vi "setValue.vi"(8 "error in (no error)":errorcluster, 10 "Time Stamp":timestamp, 11 "tBSONTimestamp in":refnum<class "tBSONTimestamp.lvclass">) -> (0 "error out":errorcluster, 3 "tBSONTimestamp out":refnum<class "tBSONTimestamp.lvclass">)   [LabVIEW 2013, in "BSON.lvlib" / "tBSONTimestamp.lvclass"]
uses:
  tBSONTimestamp.lvclass
  tBSONTimestamp.lvclass/tBSONTimestamp.ctl
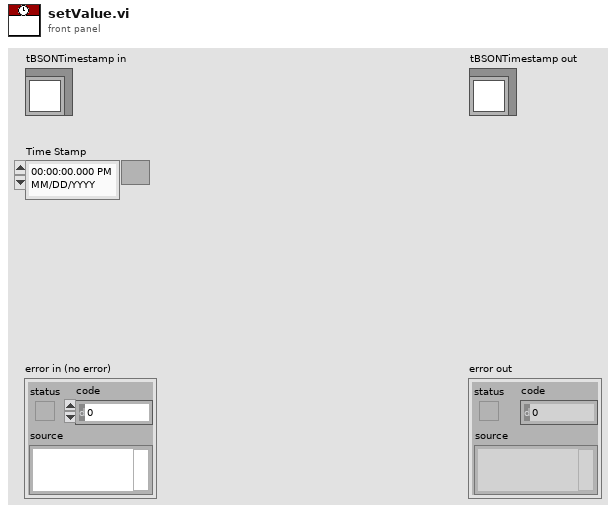
[diagram p1: front panel]
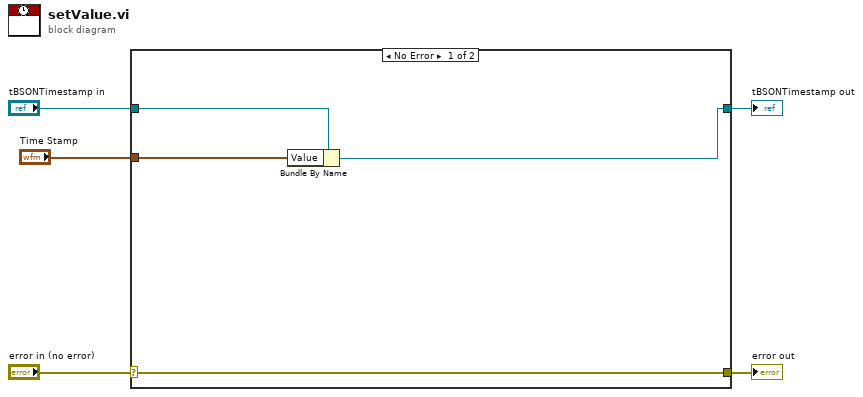
[diagram p0: block diagram]
diagram:
  n1 = case shown="No Error" "error in (no error)" {
    selector: "error in (no error)" -> [w9 w11]
    tunnel: [w9 w11] -> w4
    tunnel: [w6 w10] -> w2
    tunnel: "tBSONTimestamp in" -> [w8 w10]
    tunnel: "Time Stamp" -> [w7 _]
    frame No Error {
      n2 = Bundle By Name(cluster=w8, "Value"=w7) -> (w6:refnum<class "tBSONTimestamp.lvclass">)
    }
    frame Error {
    }
  }
  "error out" <- w4
  "tBSONTimestamp out" <- w2
